vi "load_FGM_result_data.vi"() -> (0 "QP_params":T1={"maxIter"=0, "nuN"=24, "Ns_mpc"=0, "-beta"=-0.9987945556640625, "beta+1"=1.9987945556640625}, 3 "FGM_result_data":T2)   [LabVIEW 2017, in "MPC_FXP_FGM_TestCase.lvclass"]
uses:
  MPC_FXP_FGM_TestCase.lvclass
  <vilib>/Utility/file.llb/Read Delimited Spreadsheet (DBL).vi
  fgm_result_test_data.ctl
  fpga_VIs/fixed-point/single-axis/fxp_mpc/fgm_pipiline/quadProgParams_pipe.ctl
panel:
  in  "QP_params":T1={"maxIter"=0, "nuN"=24, "Ns_mpc"=0, "-beta"=-0.9987945556640625, "beta+1"=1.9987945556640625}
  out "Ns":i16
  out "Nmpc":i16
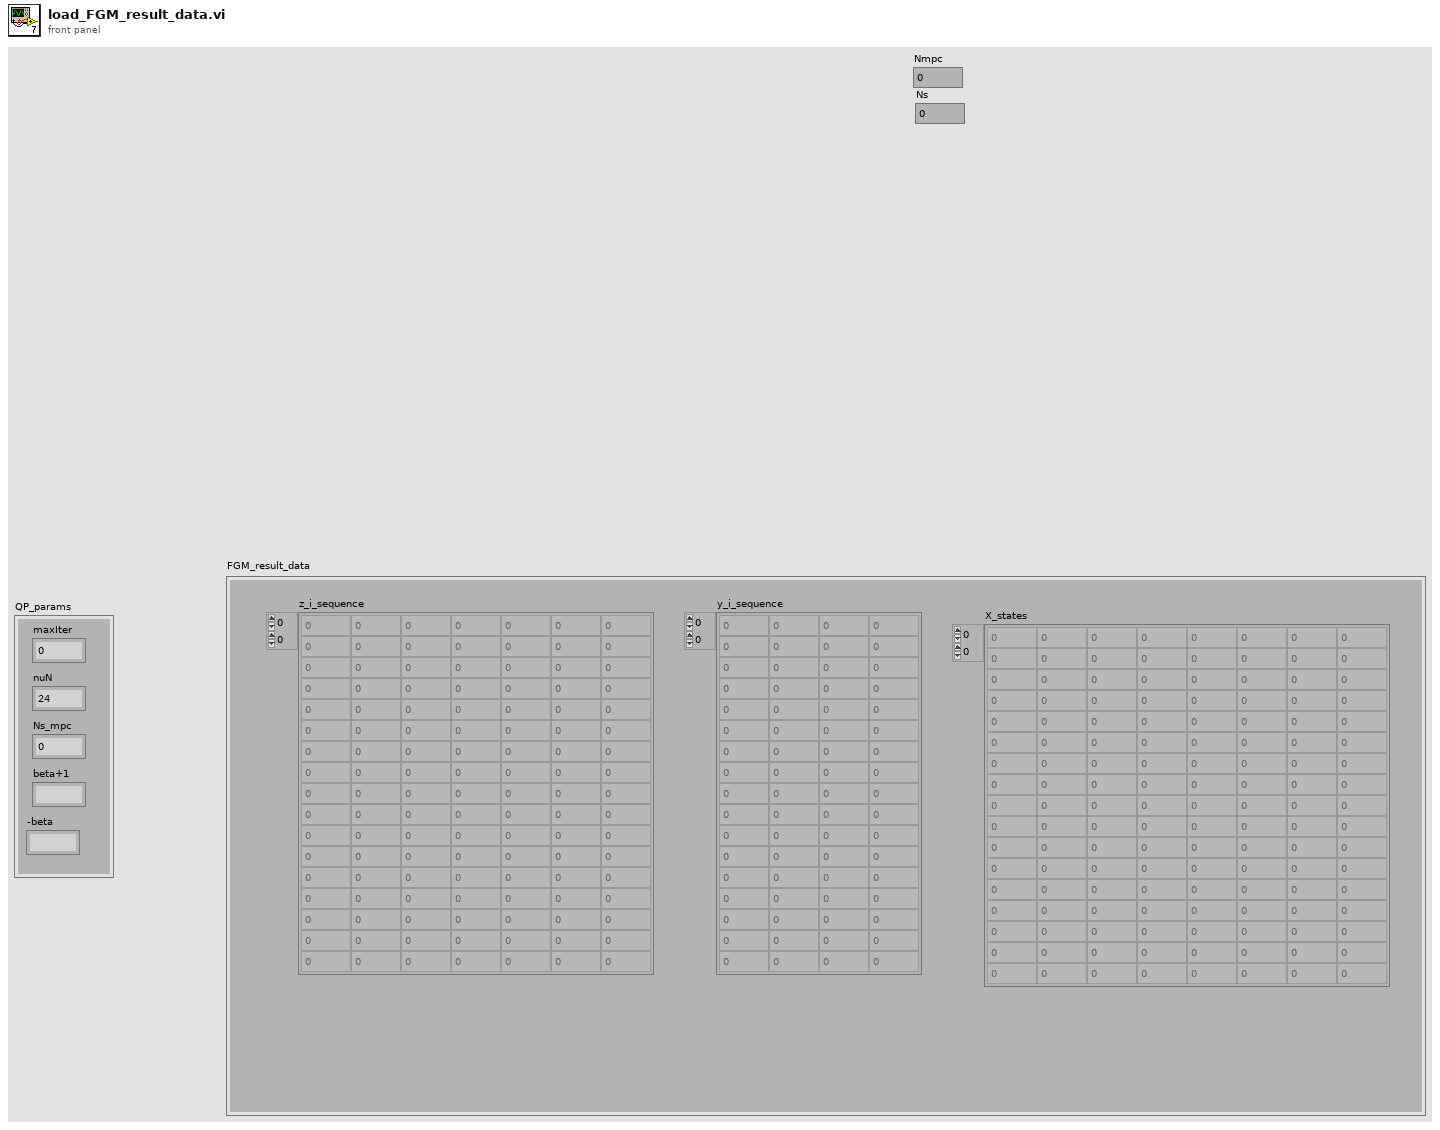
[diagram p1: front panel]
types:
  T1 = typedef "quadProgParams_pipe.ctl" = cluster{"maxIter":u16, "nuN":u16, "Ns_mpc":u16, "-beta":fxp<+/-,18,2>, "beta+1":fxp<+/-,18,2>}
  T2 = typedef "fgm_result_test_data.ctl" = cluster{"z_i_sequence":dbl[][], "y_i_sequence":dbl[][], "X_states":dbl[][]}
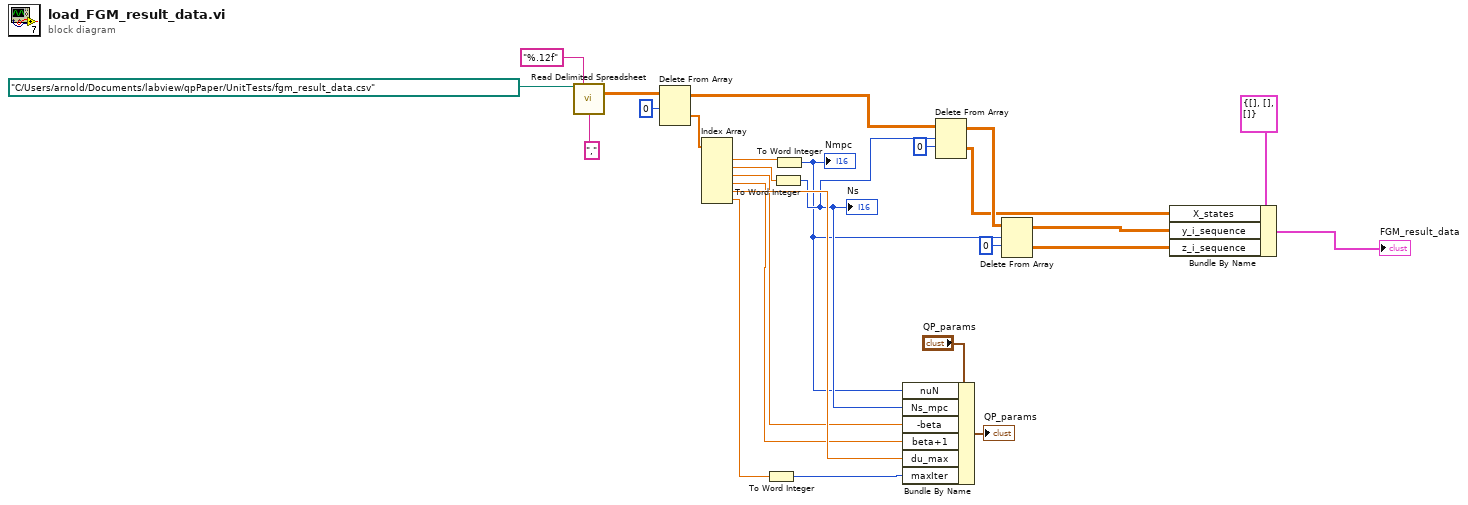
[diagram p0: block diagram]
diagram:
  n1 = call-poly <vilib>:"Read Delimited Spreadsheet.vi"("file path (dialog if empty)"=path "C:/Users/arnold/Documents/labview/qpPaper/UnitTests/fgm_result_data.csv" ("Path"), "format (%.3f)"="%.12f", "delimiter (\\t)"="," ("delimiter (\\t)")) -> ("all rows"=w23:dbl[][])  [unwired: 7 in, 5 out]
  n2 = Delete From Array(array=w23, index (row)=0) -> (deleted portion=w21:dbl[], array with subset deleted=w18:dbl[][])  [unwired: 2 in]
  n3 = Index Array(array=w21) -> (element #1=w20:dbl, element #2=w19:dbl, element #3=w4:dbl, element #4=w5:dbl, element #5=w6:dbl, element #6=w9:dbl)  [unwired: 6 in]
  n4 = To Word Integer(number=w9) -> (16bit integer=w7:i16)
  n5 = To Word Integer(number=w19) -> (16bit integer=w3:i16)
  "Ns" <- w3
  n6 = To Word Integer(number=w20) -> (16bit integer=w2:i16)
  "Nmpc" <- w2
  n7 = Bundle By Name(cluster="QP_params", "nuN"=w2, "Ns_mpc"=w3, "-beta"=w4, "beta+1"=w5, "du_max"=w6, "maxIter"=w7) -> (→"QP_params":T1)
  n8 = Delete From Array(array=w18, length=w3, index (row)=0) -> (deleted portion=w12:dbl[][], array with subset deleted=w16:dbl[][])  [unwired: 1 in]
  n9 = Delete From Array(array=w16, length=w2, index (row)=0) -> (deleted portion=w10:dbl[][], array with subset deleted=w11:dbl[][])  [unwired: 1 in]
  n10 = Bundle By Name(cluster=T2 {"z_i_sequence"=[], "y_i_sequence"=[], "X_states"=[]} ("Cluster"), "X_states"=w12, "y_i_sequence"=w11, "z_i_sequence"=w10) -> (→"FGM_result_data":T2)
